vi "initialise.vi"(8 "error in (no error)":errorcluster, 11 "GenericPlugin in":refnum<class "GenericToplevelComponent.lvclass">) -> (0 "error out":errorcluster, 3 "GenericPlugin out":refnum<class "GenericToplevelComponent.lvclass">)   [LabVIEW 2010, in "GenericToplevelComponent.lvclass"]
doc: "The dynamic dispatch-version of this VI initalises the plug-in object by allocating and initalising any dynamic resources need."
uses:
  GenericToplevelComponent.lvclass
  GenericComponent/GenericComponent/GenericComponent.lvclass
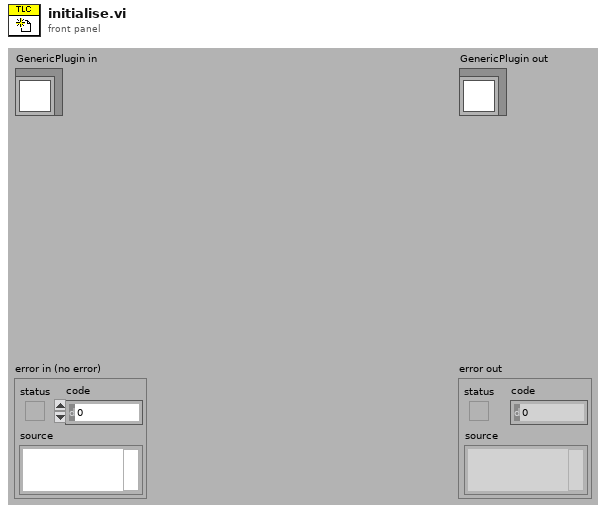
[diagram p1: front panel]
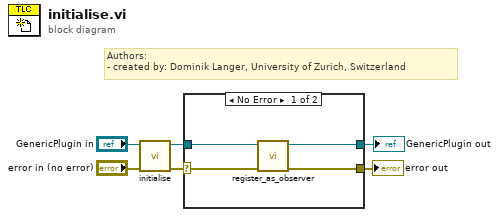
[diagram p0: block diagram]
diagram:
  # "Authors: \n- created by: Dominik Langer, University of Zurich, Switzerland"
  n1 = call-parent "initialise.vi"("error in (no error)"="error in (no error)", "GenericPlugin in"="GenericPlugin in") -> ("error out"=w1:errorcluster, "GenericPlugin out"=w3:refnum<class "GenericToplevelComponent.lvclass">)  [unwired: 8 in]
  n2 = case shown="No Error" w1 {
    selector: w1 -> [w10 w11]
    tunnel: [w9 w11] -> w4
    tunnel: w3 -> [w8 w12]
    tunnel: [w7 w12] -> w2
    frame No Error {
      n3 = call-dynamic "register_as_observer.vi"("error in (no error)"=w10, "GenericToplevelComponent in"=w8) -> ("error out"=w9:errorcluster, "GenericToplevelComponent out"=w7:refnum<class "GenericToplevelComponent.lvclass">)  [unwired: 8 in]
    }
    frame Error {
    }
  }
  "error out" <- w4
  "GenericPlugin out" <- w2
